vi "Check answer Message.vi"(4 "Error id":u8[](array[numeric]), 6 "data valid?":bool[](array[boolean]), 8 "error in (no error)":errorcluster, 11 "Siemens Ctr":T1) -> (0 "error out":errorcluster, 1 "Error message":string, 2 "Data valid?":bool, 3 "Siemens Ctr out":T1)   [LabVIEW 2014, in "Simatic S7.lvlib"]
uses:
  Simatic S7.lvlib
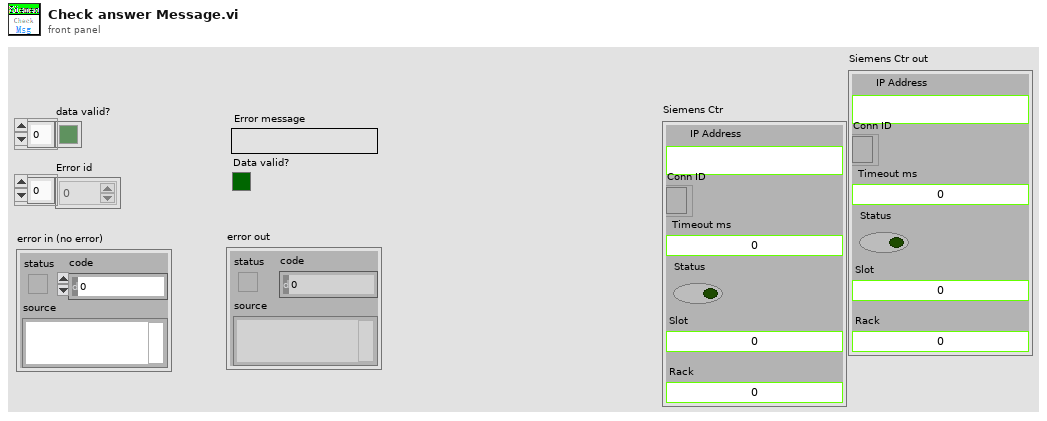
[diagram p1: front panel]
types:
  T1 = typedef "Simatic S7.lvlib/Siemens Ref.ctl" = cluster{"IP Address ":string, "Conn ID":refnum<k5>, "Timeout ms":i32, "Status":bool, "Slot":u16, "Rack":u16}
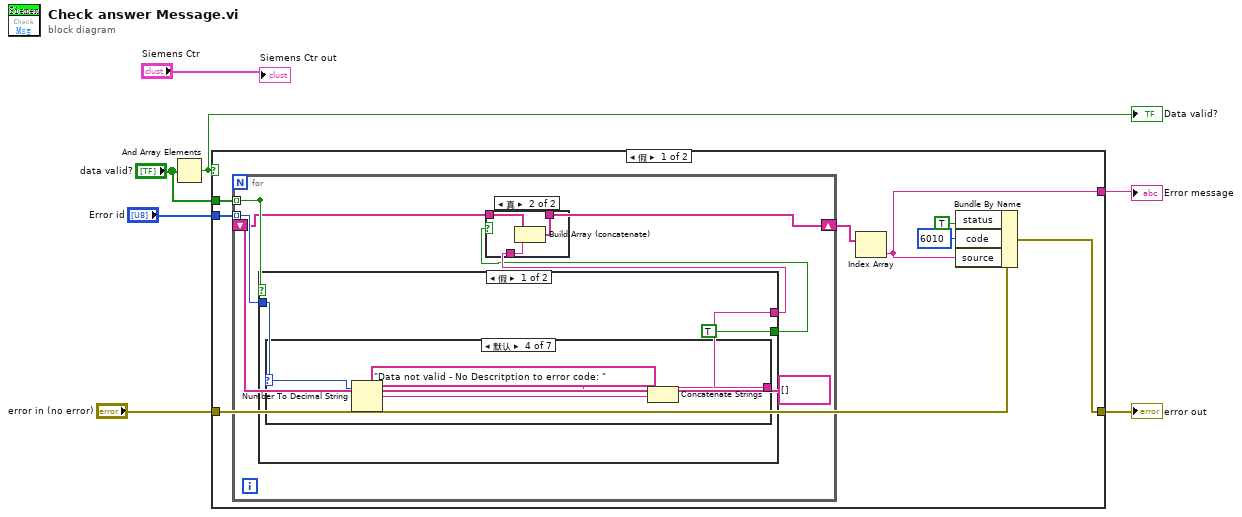
[diagram p0: block diagram]
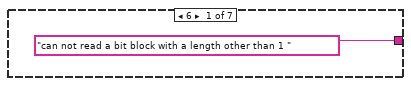
[diagram p3: hidden frame]
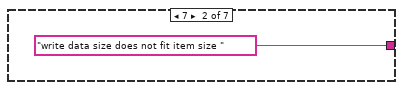
[diagram p4: hidden frame]
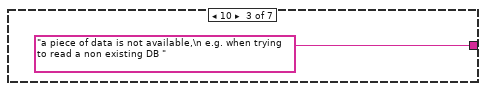
[diagram p5: hidden frame]
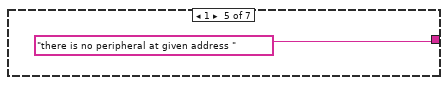
[diagram p6: hidden frame]
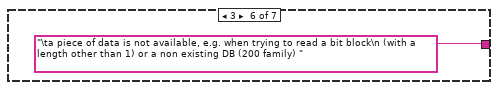
[diagram p7: hidden frame]
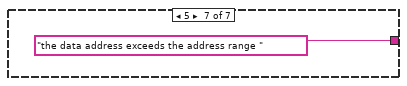
[diagram p8: hidden frame]
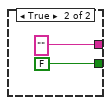
[diagram p9: hidden frame]
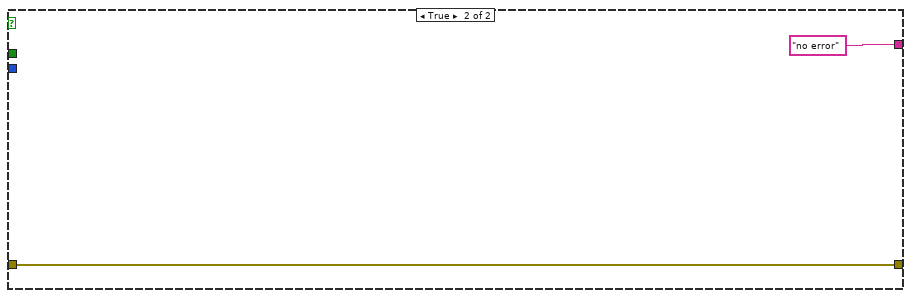
[diagram p10: hidden frame]
diagram:
  n1 = And Array Elements(Boolean array="data valid?") -> (logical AND=w7:bool)
  "Data valid?" <- w7
  n2 = case shown="假" w7 {
    tunnel: "Error id" -> [w16 _]
    tunnel: "data valid?" -> [w15 _]
    tunnel: "error in (no error)" -> [w14 w43]
    tunnel: [w10 w43] -> w3
    tunnel: [w9 "no error"] -> w2
    frame False {
      n3 = for {
        tunnel: w16 -> [w21] mode=indexing
        tunnel: [w22] -> _ mode=indexing
        tunnel: w15 -> [w22] mode=indexing
        shift-right: [w17] -> w11
        shift-left: string[] [] ("Array") -> [w18]
        n4 = case shown="假" w22 {
          tunnel: w21 -> [w29 _]
          tunnel: [w28 ""] -> w20
          tunnel: [TRUE FALSE] -> w19
          frame False {
            n5 = case shown="默认" w29 {
              selector: w29 -> [_ _ _ w36 _ _ _]
              tunnel: ["can not read a bit block with a length other than 1 " "write data size does not fit item size " "a piece of data is not available,\n e.g. when trying to read a non existing DB " w33 "there is no peripheral at given address " "\ta piece of data is not available, e.g. when trying to read a bit block\n (with a length other than 1) or a non existing DB (200 family) " "the data address exceeds the address range "] -> w28
              frame 6 {
              }
              frame 7 {
              }
              frame 10 {
              }
              frame Default {
                n6 = Number To Decimal String(number=w36) -> (decimal integer string=w34:string)  [unwired: 1 in]
                n7 = Concatenate Strings("Data not valid - No Descritption to error code: ", w34) -> (w33:string)
              }
              frame 1 {
              }
              frame 3 {
              }
              frame 5 {
              }
            }
          }
          frame True {
          }
        }
        n8 = case shown="真" w19 {
          tunnel: w18 -> [w23 w25]
          tunnel: w20 -> [_ w24]
          tunnel: [w23 w26] -> w17
          frame False {
          }
          frame True {
            n9 = Build Array (concatenate)(w25, w24) -> (w26:string[])
          }
        }
      }
      n10 = Index Array(array=w11) -> (element=w9:string)  [unwired: 1 in]
      n11 = Bundle By Name(cluster=w14, "status"=TRUE, "code"=6010, "source"=w9) -> (w10:errorcluster)
    }
    frame True {
    }
  }
  "error out" <- w3
  "Error message" <- w2
  "Siemens Ctr out" <- "Siemens Ctr"
